vi "檢測_Line_Sub.vi"(6 "邊參數":T2={"Search Direction"=0, "Edge Polarity"=0, "Kernel Size"=3, "Width"=3, "Minimum Edge Strength"=10.0} {"Minimum Edge Strength" format="%.2f"; "Width" step=2; "Kernel Size" step=2; "Edge Polarity" items=["All Edges", "Rising Edges", "Falling Edges"]; "Search Direction" items=["Left to Right", "Right to Left", "Top to Bottom", "Bottom to Top"]}, 8 "error in (no error)":errorcluster, 9 "ROI":T6, 10 "Coordinate System":T5 {"Measurement System"."Axis Reference" items=["Direct", "Indirect"]; "Measurement System"."Angle (deg)" format="%.2f"; "Measurement System"."Origin"."Y" format="%.2f"; "Measurement System"."Origin"."X" format="%.2f"; "Reference System"."Axis Reference" items=["Direct", "Indirect"]; "Reference System"."Angle (deg)" format="%.2f"; "Reference System"."Origin"."Y" format="%.2f"; "Reference System"."Origin"."X" format="%.2f"}, 11 "Image":T4) -> (0 "error out":errorcluster, 2 "線段2端點":T1 {"點2 (Pixels)"."Y" format="%.2f"; "點2 (Pixels)"."X" format="%.2f"; "點1 (Pixels)"."Y" format="%.2f"; "點1 (Pixels)"."X" format="%.2f"}, 3 "Image Out":T4)   [LabVIEW 2015]
uses:
  <vilib>/vision/Image Controls.llb/IMAQ Image.ctl
  3.Setting/Control/Setting_Control_Line Paremeter.ctl
  <vilib>/vision/Measure.llb/Edge Polarity.ctl
  <vilib>/vision/Measure.llb/Edge Options.ctl
  <vilib>/vision/NI_Vision_Development_Module.lvlib
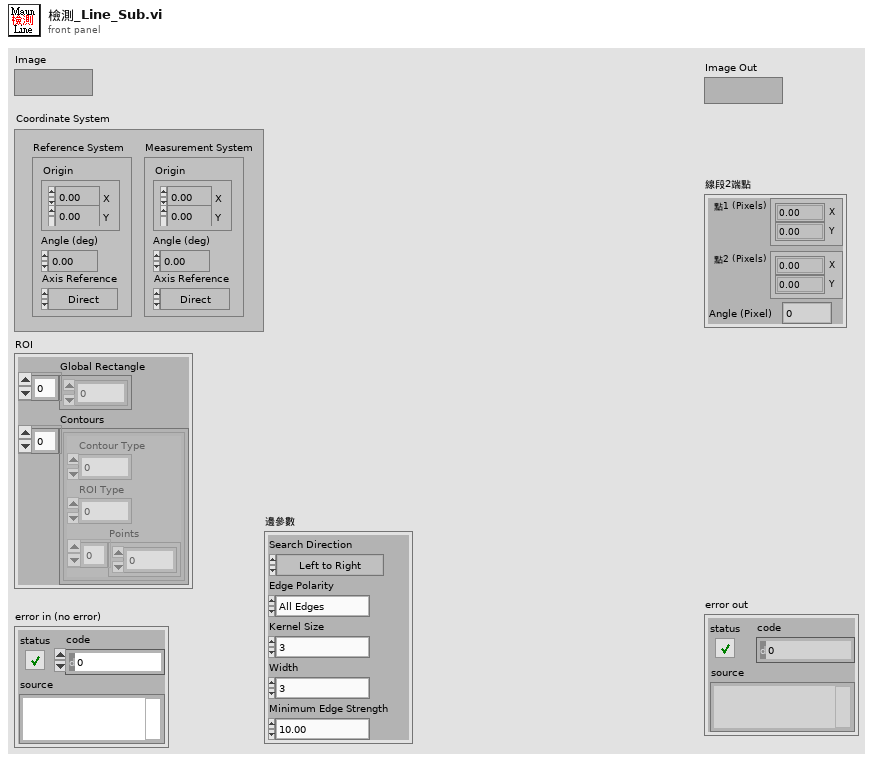
[diagram p1: front panel]
types:
  T1 = cluster{"點1 (Pixels)":cluster{"X":sgl, "Y":sgl}, "點2 (Pixels)":cluster{"X":sgl, "Y":sgl}, "Angle (Pixel)":dbl}
  T2 = typedef "Setting_Control_Line Paremeter.ctl" = cluster{"Search Direction":u32, "Edge Polarity":T3, "Kernel Size":u32, "Width":u32, "Minimum Edge Strength":sgl}
  T3 = typedef "Edge Polarity.ctl" = u32
  T4 = typedef "IMAQ Image.ctl" = refnum<image>
  T5 = typedef "IMAQ Coordinate System" = cluster{"Reference System":cluster{"Origin":cluster{"X":sgl, "Y":sgl}, "Angle (deg)":sgl, "Axis Reference":u32}, "Measurement System":cluster{"Origin":cluster{"X":sgl, "Y":sgl}, "Angle (deg)":sgl, "Axis Reference":u32}}
  T6 = cluster{"Global Rectangle":i32[], "Contours":cluster{"Contour Type":u32, "ROI Type":u32, "Points":i32[]}[]}
  T7 = typedef "Edge Options.ctl" = cluster{"Edge Polarity":T3, "Kernel Size":u32, "Width":u32, "Minimum Edge Strength":sgl, "Interpolation Type":enum32{"Zero Order", "Bilinear", "Quadratic", "Cubic", "Bilinear Fixed"}, "Data Processing Method":enum32{"Average", "Median"}}
  T8 = cluster{"Search Direction":u32, "Edge Options":T7, "Show Search Area":bool, "Show Search Lines":bool, "Show Edges Found":bool, "Show Result":bool, "Search Area Color":u32, "Search Lines Color":u32, "Edge Locations Color":u32, "Result Color":u32, "Overlay Group Name":string}
  T9 = cluster{"Point1 (Pixels)":cluster{"X":sgl, "Y":sgl}, "Point2 (Pixels)":cluster{"X":sgl, "Y":sgl}, "Point1 (Real-World)":cluster{"X":sgl, "Y":sgl}, "Point2 (Real-World)":cluster{"X":sgl, "Y":sgl}, "Angle (Pixel)":dbl, "Angle (Real-World)":dbl, "Score":dbl, "Straightness":dbl, "Average SNR (db)":dbl, "Calibration Valid":bool}[]
  T10 = cluster{"Point1 (Pixels)":cluster{"X":sgl, "Y":sgl}, "Point2 (Pixels)":cluster{"X":sgl, "Y":sgl}, "Point1 (Real-World)":cluster{"X":sgl, "Y":sgl}, "Point2 (Real-World)":cluster{"X":sgl, "Y":sgl}, "Angle (Pixel)":dbl, "Angle (Real-World)":dbl, "Score":dbl, "Straightness":dbl, "Average SNR (db)":dbl, "Calibration Valid":bool}
  T11 = cluster{"Point1 (Pixels)":cluster{"X":sgl, "Y":sgl}, "Point2 (Pixels)":cluster{"X":sgl, "Y":sgl}, "Angle (Real-World)":dbl}
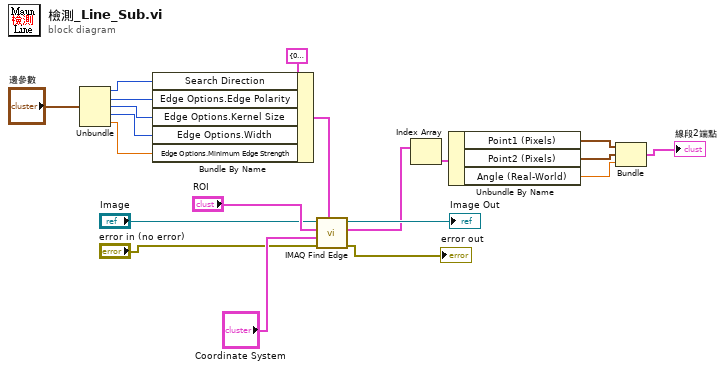
[diagram p0: block diagram]
diagram:
  n1 = Unbundle("邊參數") -> ("Search Direction"=w11:u32, "Edge Polarity"=w10:T3, "Kernel Size"=w9:u32, "Width"=w8:u32, "Minimum Edge Strength"=w7:sgl)
  n2 = Bundle By Name(cluster=T8 {"Search Direction"=0, "Edge Options"={"Edge Polarity"=0, "Kernel Size"=3, "Width"=3, "Minimum Edge Strength"=10.0, "Interpolation Type"=enum."Bilinear Fixed", "Data Processing Method"=enum."Average"}, "Show Search Area"=FALSE, "Show Search Lines"=FALSE, "Show Edges Found"=FALSE, "Show Result"=TRUE, "Search Area Color"=65280, "Search Lines Color"=255, "Edge Locations Color"=16776960, "Result Color"=16711680, "Overlay Group Name"=""} ("Options"), "Search Direction"=w11, "Edge Options.Edge Polarity"=w10, "Edge Options.Kernel Size"=w9, "Edge Options.Width"=w8, "Edge Options.Minimum Edge Strength"=w7) -> (w12:T8)
  n3 = call "IMAQ Find Edge"("Options"=w12, "error in (no error)"="error in (no error)", "Coordinate System"="Coordinate System", "ROI Descriptor"="ROI", "Image"="Image") -> ("error out"=→"error out":errorcluster, "Straight Edges"=w6:T9, "Image Out"=→"Image Out":T4)  [unwired: 3 in, 1 out]
  n4 = Index Array(array=w6) -> (element=w5:T10)  [unwired: 1 in]
  n5 = Unbundle By Name(w5) -> ("Point1 (Pixels)"=w4:cluster{"X":sgl, "Y":sgl}, "Point2 (Pixels)"=w3:cluster{"X":sgl, "Y":sgl}, "Angle (Real-World)"=w2:dbl)
  n6 = Bundle("Point1 (Pixels)"=w4, "Point2 (Pixels)"=w3, "Angle (Real-World)"=w2) -> (→"線段2端點":T11)  [unwired: 1 in]
